vi "Error Log.vi"(0 "Error log message":string, 7 "Priority":T1, 11 "error in (no error)":errorcluster, 12 "Disconnecting":bool) -> (15 "error out":errorcluster)   [LabVIEW 2011]
uses:
  Error Log - Priority.ctl
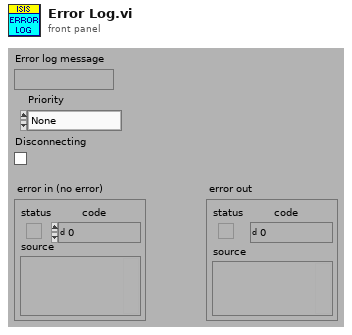
[diagram p1: front panel]
types:
  T1 = typedef "Error Log - Priority.ctl" = enum16{"None", "Log", "SECI and Log"}
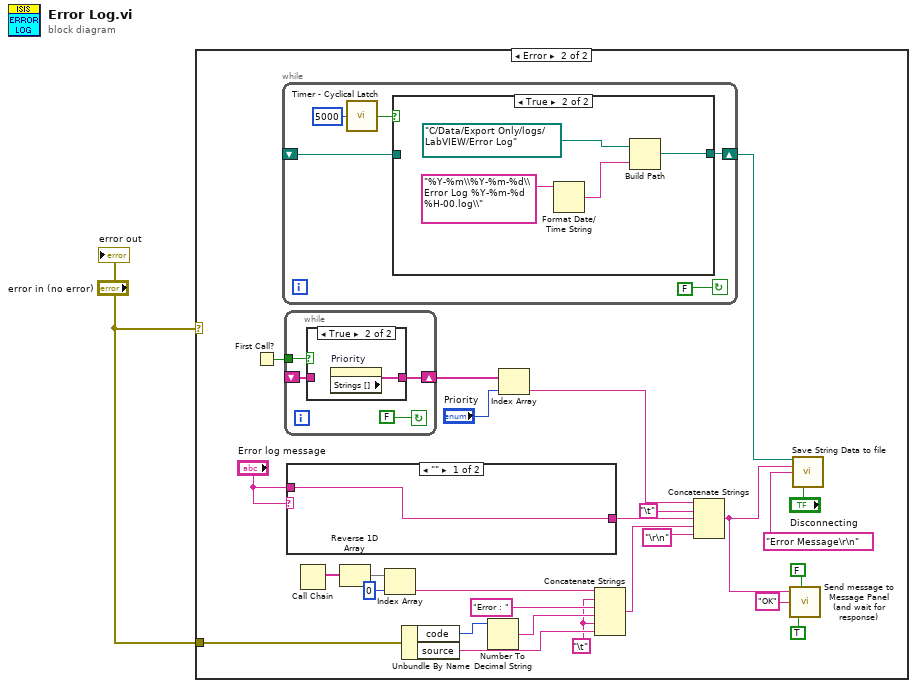
[diagram p0: block diagram]
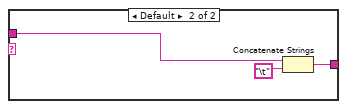
[diagram p4: hidden frame]
diagram:
  n1 = case shown="Error" "error in (no error)" {
    tunnel: "error in (no error)" -> [_ w23]
    frame No Error {
    }
    frame Error {
      w11 = "\t"
      n2 = First Call?() -> (First Call?: T/F=w10:bool)
      n3 = while {
        shift-right: [w42] -> w25
        shift-left: _ -> [w39]
        stop <- FALSE continue-if-true
        n4 = call "Timer - Cyclical Latch.vi"("Timer (msec)"=u32 5000) -> ("Timer Trigger"=w40:bool)  [unwired: 14 in]
        n5 = case shown="True" w40 {
          tunnel: [w43 w45] -> w42
          tunnel: w39 -> [w43 _]
          frame False {
          }
          frame True {
            n6 = Format Date/Time String(time format string (%c)="%Y-%m\\%Y-%m-%d\\Error Log %Y-%m-%d %H-00.log\\") -> (date/time string=w44:string)  [unwired: 2 in]
            n7 = Build Path(base path=path "C:/Data/Export Only/logs/LabVIEW/Error Log", name or relative path=w44) -> (appended path=w45:path)
          }
        }
      }
      n8 = while {
        shift-right: [w30] -> w9
        shift-left: _ -> [w29]
        tunnel: w10 -> [w28]
        stop <- FALSE continue-if-true
        n9 = case shown="True" w28 {
          tunnel: [w32 w33] -> w30
          tunnel: w29 -> [w32 _]
          frame False {
          }
          frame True {
            n10 = property on="Priority" class="Enum (strict)"() -> ("Strings []"=w33:string[])  [unwired: 2 in, 2 out]
          }
        }
      }
      n11 = case shown="\"\"" "Error log message" {
        tunnel: [w34 w37] -> w24
        tunnel: "Error log message" -> [w34 w36]
        frame "" {
        }
        frame Default {
          n12 = Concatenate Strings(w36, "\t") -> (w37:string)
        }
      }
      n13 = Call Chain() -> (call chain=w14:string[])
      n14 = Reverse 1D Array(array=w14) -> (reversed array=w15:string[])
      n15 = Index Array(array=w15, index=0) -> (element=w12:string)
      n16 = Unbundle By Name(w23) -> ("code"=w18:i32, "source"=w19:string)
      n17 = Number To Decimal String(number=w18) -> (decimal integer string=w17:string)  [unwired: 1 in]
      n18 = Index Array(array=w9, index="Priority") -> (element=w7:string)
      n19 = Concatenate Strings(w12, w11, "Error : ", w17, w11, w19) -> (w22:string)
      n20 = Concatenate Strings(w7, "\t", w24, w22, "\r\n") -> (w2:string)
      n21 = call "Send message to Message Panel (and wait for response).vi"("Prompt"=w2, "Wait for response?"=FALSE, "Yes text"="OK", "Timeout?"=TRUE) -> ()  [unwired: 1 in, 1 out]
      n22 = call "Save String Data to file.vi"("Path"=w25, "String to save"=w2, "Header"="Error Message\r\n", "Disconnecting"="Disconnecting") -> ()  [unwired: 12 in]
    }
  }
  "error out" <- "error in (no error)"
